vi "Cmd Sync with OPC and SRQ - program.vi"() -> ()   [LabVIEW 2011]
doc: "Synchronizes two commands sent to the instrument by waiting for a service request when the first operation is complete before sending the second command.\n\nThis VI is shows you how to use utility VIs to synchronize commands. Although you may run the VI interactively, it is indended to show how to combine VIs to build your application. To better understand the role of the register settings by interactively sending commands to the instrument, please refer to Example Command Sync using OPC and SRQ.vi.\n\nTo use the VI, complete the following steps: \n\n1. Select your instrument resource name from the drop-down VISA session.\n\n2. Specify the command you want to wait for in the First Command buffer.\n\n3. Specify the follow-up command or query in the Second Command/Query buffer. If the follow-up command is not a query to the instrument, set Query to False. \n\n4. Run the VI. \n\nThe VI sends the first command to the instrument, then waits on a service request. A service request occurs when the operation completes, an instrument error occurs, or the service request times out. If the operation completed successfully, the second command or query is sent to the instrument. When performing an instrument query, the Read Buffer contains the response from the instrument. \n\nNote: \nThe default commands used in this example work with the Agilent 34401A using the GPIB interface. You can use this VI with other instruments that use the IEEE 488.2 registers. However, read your instrument manual for specific details of the commands you send to the instrument."
uses:
  Low Level/Standard Event Status Indicator.ctl
  Low Level/Status Byte Indicator.ctl
panel:
  out "Actual Bytes Read":i32
  in  "Bytes to Read":i32=1024
  in  "Query":bool=TRUE
  out "Read Buffer":string
  in  "Second Command/Query":string=":FETCH?"
  out "Read SESR":T1
  in  "First Command":string=":TRIG:COUN 1;:INIT"
  in  "VISA session":refnum<visa-resource-name>
  # "This VI instructs the instrument to issue a service\nrequest when the operation associated with the\ncommand is complete."
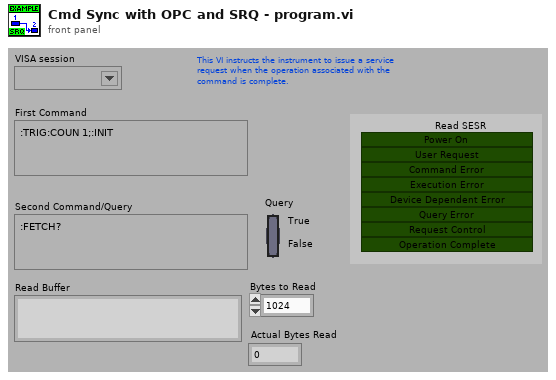
[diagram p1: front panel]
types:
  T1 = typedef "Standard Event Status Indicator.ctl" = cluster{"Operation Complete (1)":bool, "Request Control (2)":bool, "Query Error (4)":bool, "Device Dependent Error (8)":bool, "Execution Error (16)":bool, "Command Error (32)":bool, "User Request (64)":bool, "Power On (128)":bool}
  T2 = typedef "Status Byte Indicator.ctl" = cluster{"Instrument Specific (1)":bool, "Instrument Specific (2)":bool, "Instrument Specific (4)":bool, "Instrument Specific (8)":bool, "Message Available (16)":bool, "Event Status Bit (32)":bool, "Request for Service (32)":bool, "Instrument Specific (128)":bool}
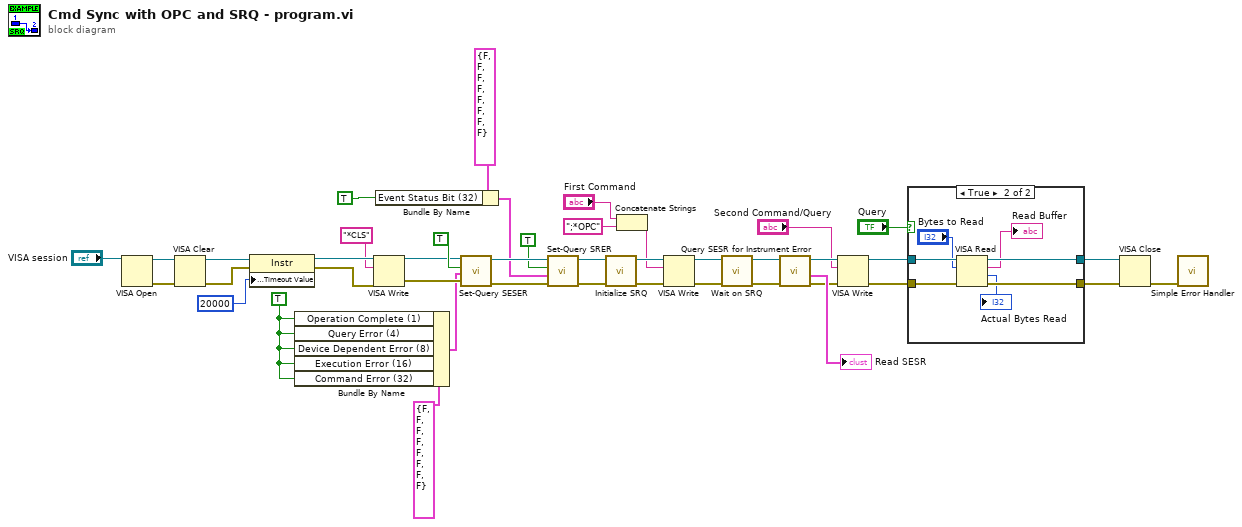
[diagram p0: block diagram]
diagram:
  w26 = TRUE ("Operation Complete")
  n1 = VISA Open(VISA resource name="VISA session") -> (VISA resource name=w4:refnum<visa-resource-name>, error out=w3:errorcluster)  [unwired: 4 in]
  n2 = VISA Clear(VISA resource name=w4, error in (no error)=w3) -> (VISA resource name out=w2:refnum<visa-resource-name>, error out=w1:errorcluster)
  n3 = property class="Instr"(reference=w2, error in=w1, "General Settings:Timeout Value"=u32 20000) -> (reference out=w36:refnum<visa-resource-name>, error out=w35:errorcluster)
  n4 = Bundle By Name(cluster=T1 {"Operation Complete (1)"=FALSE, "Request Control (2)"=FALSE, "Query Error (4)"=FALSE, "Device Dependent Error (8)"=FALSE, "Execution Error (16)"=FALSE, "Command Error (32)"=FALSE, "User Request (64)"=FALSE, "Power On (128)"=FALSE} ("Read SESR"), "Operation Complete (1)"=w26, "Query Error (4)"=w26, "Device Dependent Error (8)"=w26, "Execution Error (16)"=w26, "Command Error (32)"=w26) -> (w28:T1)
  n5 = VISA Write(VISA resource name=w36, write buffer="*CLS", error in (no error)=w35) -> (VISA resource name out=w33:refnum<visa-resource-name>, error out=w32:errorcluster)  [unwired: 1 out]
  n6 = Bundle By Name(cluster=T2 {"Instrument Specific (1)"=FALSE, "Instrument Specific (2)"=FALSE, "Instrument Specific (4)"=FALSE, "Instrument Specific (8)"=FALSE, "Message Available (16)"=FALSE, "Event Status Bit (32)"=FALSE, "Request for Service (32)"=FALSE, "Instrument Specific (128)"=FALSE} ("Read SBR"), "Event Status Bit (32)"=TRUE ("Instrument Specific")) -> (w27:T2)
  n7 = call "Set-Query SESER.vi"("error in (no error)"=w32, "Enable SESER"=w28, "Enable Mask (T)"=TRUE ("Enable Mask"), "VISA session"=w33) -> ("error out"=w39:errorcluster, "dup VISA session"=w40:refnum<visa-resource-name>)  [unwired: 5 in, 1 out]
  n8 = call "Set-Query SRER.vi"("error   in (no error)"=w39, "Enable SRER"=w27, "Enable Mask (T)"=TRUE ("function"), "VISA session"=w40) -> ("error out"=w31:errorcluster, "dup VISA session"=w29:refnum<visa-resource-name>)  [unwired: 5 in, 1 out]
  n9 = call "Initialize SRQ.vi"("error in"=w31, "dup VISA session"=w29) -> ("error out (no error)"=w18:errorcluster, "dup VISA session"=w19:refnum<visa-resource-name>)  [unwired: 8 in]
  n10 = Concatenate Strings("First Command", ";*OPC" ("string")) -> (w17:string)
  n11 = VISA Write(VISA resource name=w19, write buffer=w17, error in (no error)=w18) -> (VISA resource name out=w20:refnum<visa-resource-name>, error out=w21:errorcluster)  [unwired: 1 out]
  n12 = call "Wait on SRQ.vi"("error in (no error)"=w21, "VISA session"=w20) -> ("error out"=w15:errorcluster, "dup VISA session"=w16:refnum<visa-resource-name>)  [unwired: 8 in]
  n13 = call "Query SESR for Instrument Error.vi"("error in (no error)"=w15, "VISA session"=w16) -> ("error out"=w13:errorcluster, "Read SESR"=→"Read SESR":T1, "dup VISA session"=w14:refnum<visa-resource-name>)  [unwired: 7 in]
  n14 = VISA Write(VISA resource name=w14, write buffer="Second Command/Query", error in (no error)=w13) -> (VISA resource name out=w9:refnum<visa-resource-name>, error out=w8:errorcluster)  [unwired: 1 out]
  n15 = case shown="True" "Query" {
    tunnel: w9 -> [w44 w51]
    tunnel: w8 -> [w43 w50]
    tunnel: [w44 w49] -> w7
    tunnel: [w43 w48] -> w6
    frame False {
    }
    frame True {
      n16 = VISA Read(VISA resource name=w51, byte count="Bytes to Read", error in (no error)=w50) -> (VISA resource name out=w49:refnum<visa-resource-name>, read buffer=→"Read Buffer":string, return count=→"Actual Bytes Read":u32, error out=w48:errorcluster)
    }
  }
  n17 = VISA Close(VISA resource name=w7, error in (no error)=w6) -> (error out=w30:errorcluster)
  n18 = call <vilib>:"Simple Error Handler.vi"("error in (no error)"=w30) -> ()  [unwired: 4 in, 5 out]
